vi "读取数据.vi"(7 "工作表名称":string="Sheet1", 8 "错误输入（无错误）":errorcluster, 11 "引用簇":T1) -> (0 "错误输出":errorcluster, 3 "引用簇输出":T1, 5 "Excel数据":string[][](array[string]))   [LabVIEW 2020, in "OperateExcel.lvlib"]
uses:
  OperateExcel.lvlib
  <vilib>/ErrorRing/Error Ring.xnode
  <vilib>/Utility/error.llb/Error Cluster From Error Code.vi
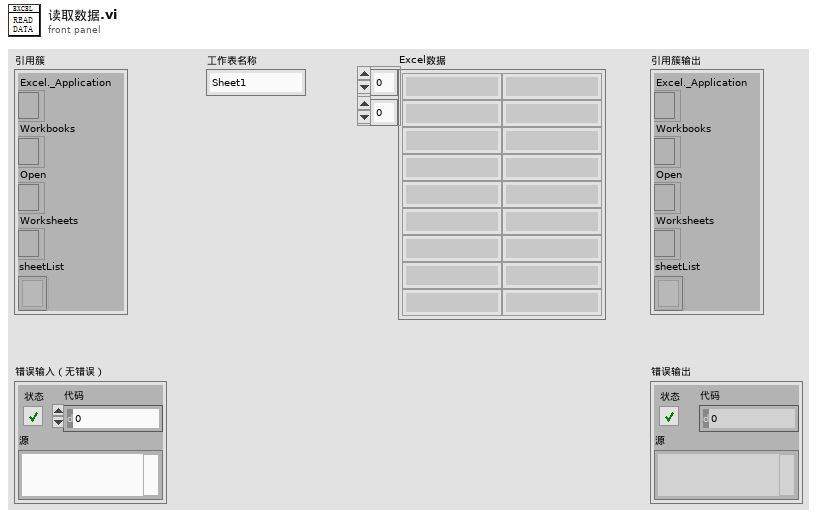
[diagram p1: front panel]
types:
  T1 = typedef "OperateExcel.lvlib/引用簇.ctl" = cluster{"Excel._Application":refnum<k7>, "Workbooks":refnum<k7>, "Open":refnum<k7>, "Worksheets":refnum<k7>, "sheetList":refnum<k7>[]}
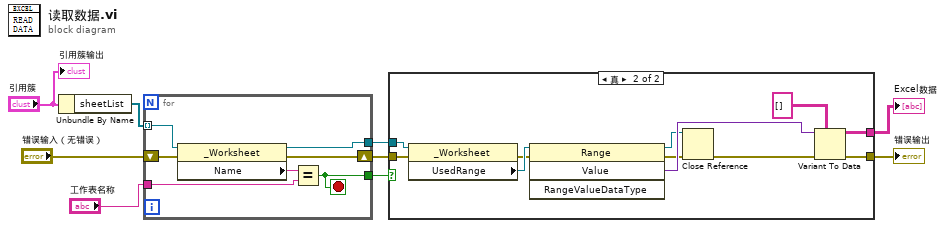
[diagram p0: block diagram]
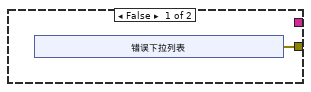
[diagram p2: hidden frame]
diagram:
  n1 = Unbundle By Name("引用簇") -> ("sheetList"=w7:refnum<k7>[])
  n2 = for {
    tunnel: w7 -> [w16] mode=indexing
    tunnel: "工作表名称" -> [w12]
    tunnel: [w15] -> w3
    shift-right: [w13] -> w4
    shift-left: "错误输入（无错误）" -> [w14]
    tunnel: [w10] -> w1
    stop <- w10 stop-if-true
    n3 = property class="_Worksheet"(reference=w16, error in=w14) -> (reference out=w15:refnum<k7>, error out=w13:errorcluster, "Name"=w11:string)
    n4 = Equal?(x=w11, y=w12) -> (x = y?=w10:bool)
  }
  n5 = case shown="真" w1 {
    tunnel: w4 -> [_ w32]
    tunnel: [w17 w31] -> w8
    tunnel: [_ w30] -> w9
    tunnel: w3 -> [_ w28]
    frame False {
      n6 = xnode "错误下拉列表"() -> ("错误输出"=w17:errorcluster)
    }
    frame True {
      n7 = property class="_Worksheet"(reference=w28, error in=w32) -> (error out=w26:errorcluster, "UsedRange"=w27:refnum<k7>)  [unwired: 1 out]
      n8 = invoke class="Range" method="Value"(reference=w27, error in=w26) -> (reference out=w25:refnum<k7>, error out=w24:errorcluster, "Value"=w29:variant)  [unwired: 2 in, 1 out]
      n9 = Close Reference(reference=w25, error in (no error)=w24) -> (error out=w23:errorcluster)
      n10 = Variant To Data(error in=w23, type=string[][] [], Variant=w29) -> (data=w30:string[][], error out=w31:errorcluster)
    }
  }
  "错误输出" <- w8
  "Excel数据" <- w9
  "引用簇输出" <- "引用簇"
